vi "Split 2D Array 2012 NIVerified.vi"(10 "index (row)":i32, 11 "Input array":string[][](array[string])) -> (2 "Lower":string[][](array[string]), 3 "Upper":string[][](array[string]))   [LabVIEW 2012]
doc: "VI receives a 2D array of strings and splits it into an Upper and Lower arrays. The split happens at the row index specified.\nIt can be easily modified to accept arrays from other data types."
panel:
  # "Overview: Demonstrate the use of Index Array functions to split a 2D array at a specified index. \nRequirements: Labview Full Development System\nInstructions:\n1. Input a 2D array.\n2. Run the VI."
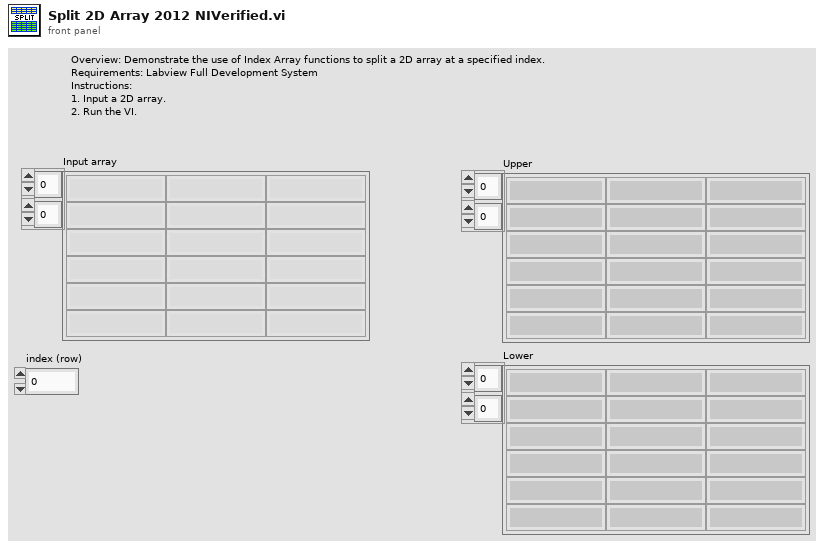
[diagram p1: front panel]
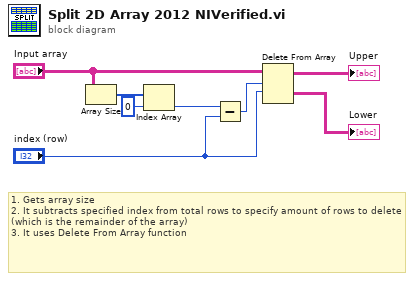
[diagram p0: block diagram]
diagram:
  # "1. Gets array size\n2. It subtracts specified index from total rows to specify amount of rows to delete (which is the remainder of the array)\n3. It uses Delete From Array function"
  n1 = Array Size(array="Input array") -> (size(s)=w6:i32[])
  n2 = Index Array(array=w6, index=0) -> (element=w2:i32)
  n3 = Subtract(x=w2, y="index (row)") -> (x-y=w4:i32)
  n4 = Delete From Array(array="Input array", length=w4, index (row)="index (row)") -> (deleted portion=→"Lower":string[][], array with subset deleted=→"Upper":string[][])  [unwired: 1 in]
